vi "FGV EX 2 SUBVI.vi"(7 "Enum":enum16{"Write Data", "Read Data"}(ring), 8 "error in (no error)":errorcluster, 11 "input in":dbl) -> (3 "input out":dbl)   [LabVIEW 2022 SP3]
panel:
  out "error out":errorcluster
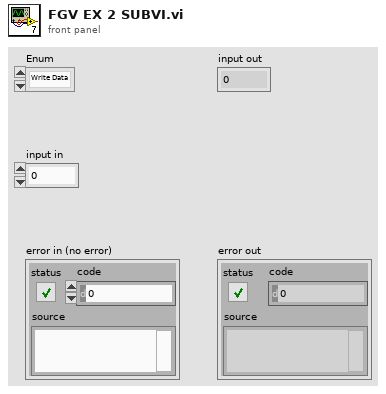
[diagram p1: front panel]
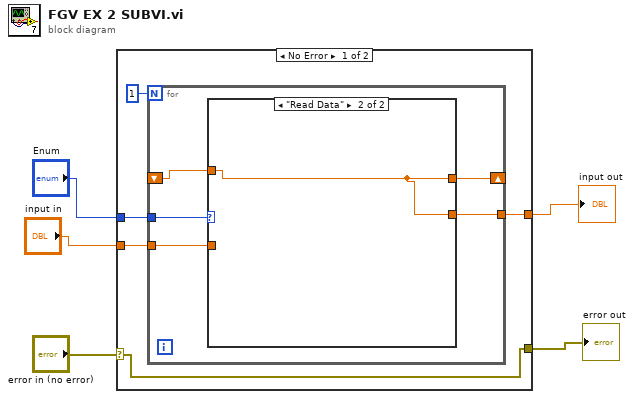
[diagram p0: block diagram]
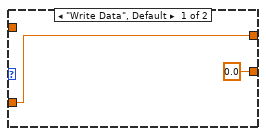
[diagram p2: hidden frame]
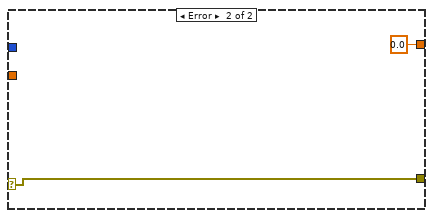
[diagram p3: hidden frame]
diagram:
  n1 = case shown="No Error" "error in (no error)" {
    selector: "error in (no error)" -> [w7 w20]
    tunnel: [w7 w20] -> w2
    tunnel: "Enum" -> [w9 _]
    tunnel: "input in" -> [w8 _]
    tunnel: [w6 0.0 ("input")] -> w5
    frame No Error {
      n2 = for {
        N: 1 -> [_]
        tunnel: w9 -> [w15]
        tunnel: w8 -> [w14]
        shift-right: [w12] -> _
        shift-left: _ -> [w13]
        tunnel: [w11] -> w6
        n3 = case shown="\"Read Data\"" w15 {
          tunnel: w14 -> [w17 _]
          tunnel: w13 -> [_ w18]
          tunnel: [w17 w18] -> w12
          tunnel: [0.0 ("input") w18] -> w11
          frame "Write Data", Default {
          }
          frame "Read Data" {
          }
        }
      }
    }
    frame Error {
    }
  }
  "input out" <- w5
  "error out" <- w2
